vi "set_data_for_channel.vi"(8 "error in (no error)":errorcluster, 10 "data":dbl[](array[numeric]), 11 "GenericWriteSignals in":refnum<class "SignalWriterMH110203USBStepperMotor.lvclass">) -> (0 "error out":errorcluster, 3 "GenericWriteSignals out":refnum<class "SignalWriterMH110203USBStepperMotor.lvclass">)   [LabVIEW 2010, in "SignalWriterMH110203USBStepperMotor.lvclass"]
uses:
  SignalWriterMH110203USBStepperMotor.lvclass
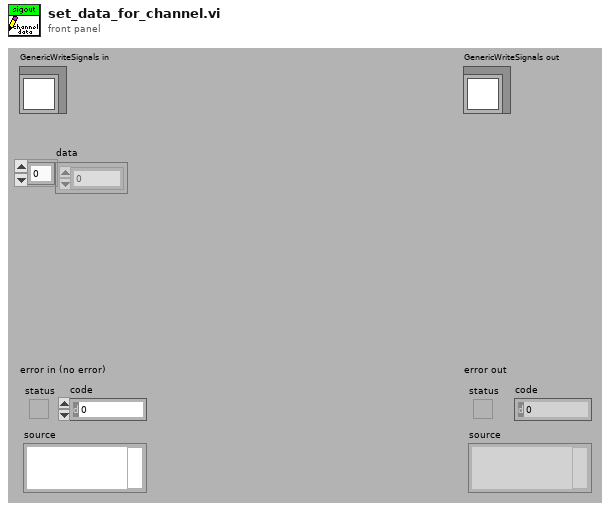
[diagram p1: front panel]
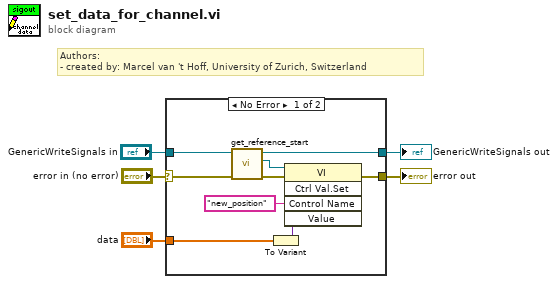
[diagram p0: block diagram]
diagram:
  # "Authors: \n- created by: Marcel van 't Hoff, University of Zurich, Switzerland"
  n1 = case shown="No Error" "error in (no error)" {
    selector: "error in (no error)" -> [w8 w16]
    tunnel: [w7 w16] -> w4
    tunnel: "GenericWriteSignals in" -> [w10 w15]
    tunnel: "data" -> [w6 _]
    tunnel: [w9 w15] -> w1
    frame No Error {
      n2 = call-dynamic "get_reference_start.vi"("error in (no error)"=w8, "SignalWriterMH110203USBStepperMotor in"=w10) -> ("error out"=w13:errorcluster, "vi reference"=w14:refnum<vi>, "SignalWriterMH110203USBStepperMotor out"=w9:refnum<class "SignalWriterMH110203USBStepperMotor.lvclass">)  [unwired: 7 in]
      n3 = To Variant(anything=w6) -> (Variant=w12:variant)
      n4 = invoke class="VI" method="Ctrl Val.Set"(reference=w14, error in=w13, "Control Name"="new_position", "Value"=w12) -> (error out=w7:errorcluster)  [unwired: 1 in, 4 out]
    }
    frame Error {
    }
  }
  "error out" <- w4
  "GenericWriteSignals out" <- w1
